vi "Lifetime batch.vi"(5 "Collection Time (seconds)":dbl=4.0, 6 "File Path Control":path, 7 "Array - Numeric":dbl[][](array[numeric]), 8 "Z Position":dbl, 9 "RS232 settings":cluster{"Portnumber":i32, "Baudrate":u16}={"Portnumber"=12, "Baudrate"=5} {"Portnumber" items=["COM1", "COM2", "COM3", "COM4", "COM5", "COM6", "COM7", "COM8", "COM9", "COM10", "COM11", "COM12", "COM13", "COM14", "COM15", "COM16", "COM17", "COM18", "COM19", "COM20", "COM21", "COM22", "COM23", "COM24", "COM25", "COM26", "COM27", "COM28", "COM29", "COM30"]; "Baudrate" items=["9600", "14400", "19200", "38400", "57600", "115200"]}, 10 "Y Parameters":T1={"Number of Y Steps"=200, "Max Y (V)"=2.0, "Min Y (V)"=-2.0}, 11 "X Parameters":T2={"Number of X Steps"=200, "Max X (V)"=2.0, "Min X (V)"=-2.0}) -> (0 "Z Position 2":dbl)   [LabVIEW 2012]
uses:
  SPCM files/Global FIFO variabls.vi
panel:
  out "Numeric":i32
  in  "stop":bool
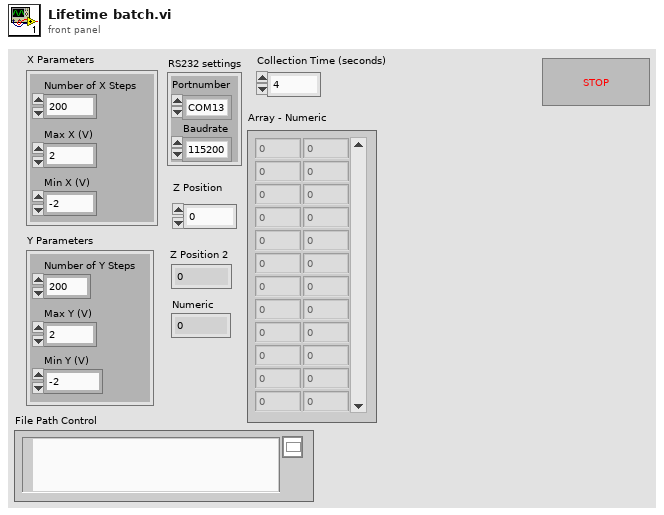
[diagram p1: front panel]
types:
  T1 = cluster{"Number of Y Steps":i32, "Max Y (V)":dbl, "Min Y (V)":dbl}
  T2 = cluster{"Number of X Steps":i32, "Max X (V)":dbl, "Min X (V)":dbl}
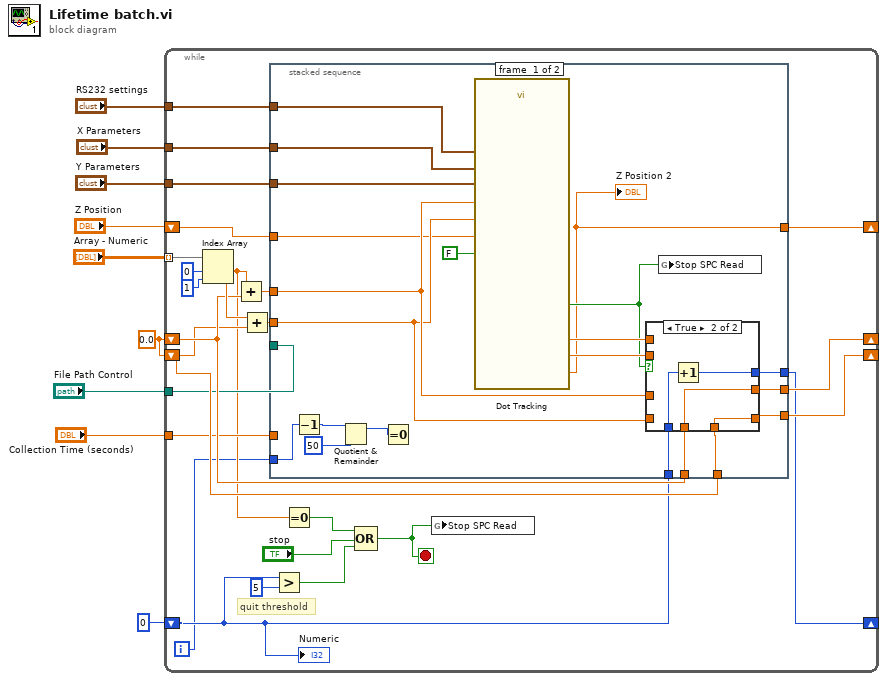
[diagram p0: block diagram]
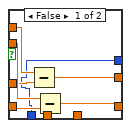
[diagram p2: hidden frame]
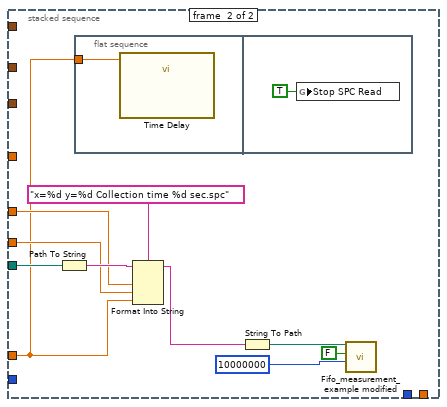
[diagram p3: hidden frame]
diagram:
  w5 = 0.0
  n1 = while {
    tunnel: "RS232 settings" -> [w35]
    tunnel: "X Parameters" -> [w34]
    tunnel: "Y Parameters" -> [w33]
    tunnel: "Array - Numeric" -> [w32] mode=indexing
    shift-right: [w26] -> _
    shift-left: w5 -> [w23]
    shift-right: [w25] -> _
    shift-left: w5 -> [w22]
    tunnel: "File Path Control" -> [w21]
    tunnel: "Collection Time (seconds)" -> [w20]
    shift-right: [w15] -> _
    shift-left: "Z Position" -> [w24]
    shift-right: [w14] -> _
    shift-left: 0 -> [w13]
    i -> [w10]
    stop <- w16 stop-if-true
    # "quit threshold"
    n2 = Index Array(array=w32, index #1=0 ("index (row)"), index #2=1 ("index (row)")) -> (element #1=w19:dbl, element #2=w28:dbl)
    n3 = Add(x=w19, y=w23) -> (x+y=w29:dbl)
    n4 = Add(x=w28, y=w22) -> (x+y=w27:dbl)
    n5 = stacked-sequence {
      tunnel: w35 -> [w56 _]
      tunnel: w34 -> [w55 _]
      tunnel: w33 -> [w54 _]
      tunnel: w29 -> [w51 w74]
      tunnel: w27 -> [w50 w73]
      tunnel: [w49 _] -> w26
      tunnel: [w48 _] -> w25
      tunnel: w24 -> [w47 _]
      tunnel: w23 -> [w46 _]
      tunnel: w22 -> [w45 _]
      tunnel: w21 -> [_ w76]
      tunnel: w20 -> [_ w68]
      tunnel: [w43 _] -> w15
      tunnel: w13 -> [w42 _]
      tunnel: [w41 _] -> w14
      tunnel: w10 -> [w40 _]
      frame #0 {
        n6 = Decrement(x=w40) -> (x-1=w39:i32)
        n7 = Quotient & Remainder(x=w39, y=50) -> (x-y*floor(x/y)=w37:i32)  [unwired: 1 out]
        n8 = Equal To 0?(x=w37) -> ()  [unwired: 1 out]
        n9 = call "Dot Tracking.vi"("X"=w55, "Y Parameters"=w54, "RS232 settings"=w56, "X Pos"=w51, "Y pos"=w50, "Z Pos"=w47, "Z-track?"=FALSE) -> ("X Position"=w53:dbl, "Y Position"=w52:dbl, "Z Position"=w43:dbl, "Gave up?"=w44:bool)  [unwired: 2 in, 3 out]
        "Z Position 2" <- w43
        n10 = case shown="True" w44 {
          tunnel: w53 -> [w63 _]
          tunnel: w52 -> [w62 _]
          tunnel: w51 -> [w61 _]
          tunnel: w50 -> [w60 _]
          tunnel: [w59 w67] -> w49
          tunnel: [w58 w66] -> w48
          tunnel: w46 -> [_ w67]
          tunnel: w45 -> [_ w66]
          tunnel: w42 -> [w57 w65]
          tunnel: [w57 w64] -> w41
          frame False {
            n11 = Subtract(x=w63, y=w61) -> (x-y=w59:dbl)
            n12 = Subtract(x=w62, y=w60) -> (x-y=w58:dbl)
          }
          frame True {
            n13 = Increment(x=w65) -> (x+1=w64:i32)
          }
        }
        n14 = global write "Global FIFO variabls.vi" "Stop SPC Read"(w44) -> ()
      }
      frame #1 {
        n15 = Path To String(path=w76) -> (string=w75:string)
        n16 = flat-sequence {
          tunnel: w68 -> [w78]
          frame #0 {
            n17 = call "Time Delay"("Delay Time (s)"=w78) -> ()  [unwired: 10 in, 1 out]
          }
          frame #1 {
            n18 = global write "Global FIFO variabls.vi" "Stop SPC Read"(TRUE ("Stop SPC Read")) -> ()
          }
        }
        n19 = Format Into String(format string="x=%d y=%d Collection time %d sec.spc", initial string=w75, w74, w73, w68) -> (resulting string=w71:string)  [unwired: 1 in, 1 out]
        n20 = String To Path(string=w71) -> (path=w70:path)
        n21 = call "Fifo_measurement_example modified.vi"("Required No of photons"=u32 10000000, "append to file? (new file:F)"=FALSE, "file path (dialog if empty)"=w70) -> ()  [unwired: 2 in, 1 out]
      }
    }
    n22 = Greater?(x=w13, y=5) -> (0:w11:bool)
    n23 = Equal To 0?(x=w19) -> (x = 0?=w18:bool)
    n24 = Compound Arithmetic op=OR(w18, "stop", w11) -> (w16:bool)
    n25 = global write "Global FIFO variabls.vi" "Stop SPC Read"(w16) -> ()
    "Numeric" <- w13
  }
